vi "GetRangeAndUnits.vi"(0 "Handle":u64, 1 "Controller Channel":i64) -> (7 "FT_Status":u64(ring) items=["FT_OK", "FT_INVALID_HANDLE", "FT_DEVICE_NOT_FOUND", "FT_DEVICE_NOT_OPENED", "FT_IO_ERROR", "FT_INSUFFICIENT_RESOURCES", "FT_INVALID_PARAMETER", "FT_INVALID_BAUD_RATE", "FT_DEVICE_NOT_OPENED_FOR_ERASE", "FT_DEVICE_NOT_OPENED_FOR_WRITE", "FT_FAILED_TO_WRITE_DEVICE", "FT_EEPROM_READ_FAILED", "FT_EEPROM_WRITE_FAILED", "FT_EEPROM_ERASE_FAILED", "FT_EEPROM_NOT_PRESENT", "FT_EEPROM_NOT_PROGRAMMED", "FT_INVALID_ARGS", "FT_NOT_SUPPORTED", "FT_OTHER_ERROR"], 9 "Range":i32, 10 "Range Units":string)   [LabVIEW 2018]
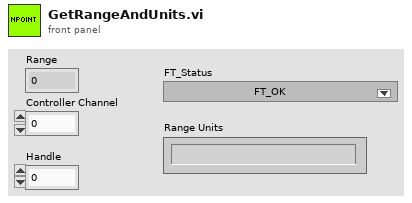
[diagram p1: front panel]
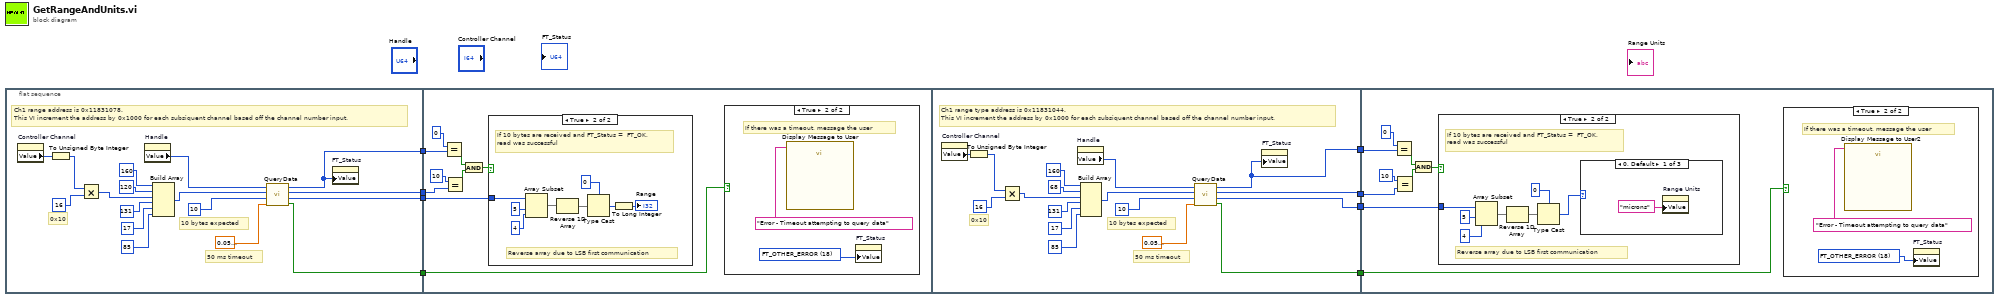
[diagram p0: block diagram]
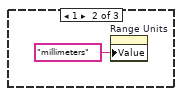
[diagram p6: hidden frame]
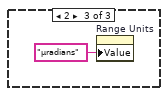
[diagram p7: hidden frame]
diagram:
  n1 = flat-sequence {
    tunnel: [w16] -> w8
    tunnel: [w15] -> w7
    tunnel: [w14] -> w6
    tunnel: [w13] -> w5
    tunnel: w8 -> [w34]
    tunnel: w7 -> [w32]
    tunnel: w6 -> [w31]
    tunnel: w5 -> [w29]
    tunnel: [w48] -> w4
    tunnel: [w52] -> w3
    tunnel: [w51] -> w2
    tunnel: [w50] -> w1
    tunnel: w4 -> [w65]
    tunnel: w3 -> [w62]
    tunnel: w2 -> [w64]
    tunnel: w1 -> [w63]
    frame #0 {
      # "10 bytes expected"
      # "50 ms timeout"
      # "Ch1 range address is 0x11831078.\nThis VI increment the address by 0x1000 for each subsiquent channel based off the channel number input."
      # "0x10"
      n2 = property on="Controller Channel" class="DigNum (strict)"() -> ("Value"=w11:i64)  [unwired: 2 in, 2 out]
      n3 = To Unsigned Byte Integer(number=w11) -> (unsigned 8bit integer=w9:u8)
      n4 = Multiply(x=w9, y=u8 16) -> (x*y=w12:u8)
      n5 = property on="Handle" class="DigNum (strict)"() -> ("Value"=w10:u64)  [unwired: 2 in, 2 out]
      n6 = Build Array(u8 160 ("element"), u8 120 ("element"), w12, u8 131 ("element"), u8 17 ("element"), u8 85 ("element")) -> (w19:u8[])
      n7 = call "QueryData.vi"("TimeoutLengthSeconds"=sgl 0.05, "NumBytesExpected"=u64 10, "Message"=w19, "Handle"=w10) -> ("Timeout"=w14:bool, "Return Array"=w15:u8[], "Bytes Read"=w16:u64, "FT_Status"=w13:u64)  [unwired: 4 in]
      n8 = property on="FT_Status" class="Ring (strict)"("Value"=w13) -> ()  [unwired: 2 in, 2 out]
    }
    frame #1 {
      n9 = Equal?(x=u64 0, y=w29) -> (x = y?=w27:bool)
      n10 = Equal?(x=u64 10, y=w34) -> (x = y?=w28:bool)
      n11 = And(x=w27, y=w28) -> (x .and. y?=w26:bool)
      n12 = case shown="True" w26 {
        tunnel: w32 -> [_ w44]
        frame False {
        }
        frame True {
          # "Reverse array due to LSB first communication"
          # "If 10 bytes are received and FT_Status =  FT_OK,\nread was successful"
          n13 = Array Subset(array=w44, index=5, length=4) -> (w40:u8[])
          n14 = Reverse 1D Array(array=w40) -> (reversed array=w39:u8[])
          n15 = Type Cast(type=0, x=w39) -> (*(type *) &x=w38:i32)
          n16 = To Long Integer(number=w38) -> (32bit integer=→"Range":i32)
        }
      }
      n17 = case shown="True" w31 {
        frame False {
        }
        frame True {
          w35 = u64 18 items=["FT_OK", "FT_INVALID_HANDLE", "FT_DEVICE_NOT_FOUND", "FT_DEVICE_NOT_OPENED", "FT_IO_ERROR", "FT_INSUFFICIENT_RESOURCES", "FT_INVALID_PARAMETER", "FT_INVALID_BAUD_RATE", "FT_DEVICE_NOT_OPENED_FOR_ERASE", "FT_DEVICE_NOT_OPENED_FOR_WRITE", "FT_FAILED_TO_WRITE_DEVICE", "FT_EEPROM_READ_FAILED", "FT_EEPROM_WRITE_FAILED", "FT_EEPROM_ERASE_FAILED", "FT_EEPROM_NOT_PRESENT", "FT_EEPROM_NOT_PROGRAMMED", "FT_INVALID_ARGS", "FT_NOT_SUPPORTED", "FT_OTHER_ERROR"] ("FT_Status")
          # "If there was a timeout, message the user"
          n18 = call "Display Message to User"("Message"="Error - Timeout attempting to query data") -> ()  [unwired: 9 in, 2 out]
          n19 = property on="FT_Status" class="Ring (strict)"("Value"=w35) -> ()  [unwired: 2 in, 2 out]
        }
      }
    }
    frame #2 {
      # "10 bytes expected"
      # "50 ms timeout"
      # "Ch1 range type address is 0x11831044.\nThis VI increment the address by 0x1000 for each subsiquent channel based off the channel number input."
      # "0x10"
      n20 = property on="Controller Channel" class="DigNum (strict)"() -> ("Value"=w47:i64)  [unwired: 2 in, 2 out]
      n21 = To Unsigned Byte Integer(number=w47) -> (unsigned 8bit integer=w45:u8)
      n22 = Multiply(x=w45, y=u8 16) -> (x*y=w49:u8)
      n23 = property on="Handle" class="DigNum (strict)"() -> ("Value"=w46:u64)  [unwired: 2 in, 2 out]
      n24 = Build Array(u8 160 ("element"), u8 68 ("element"), w49, u8 131 ("element"), u8 17 ("element"), u8 85 ("element")) -> (w55:u8[])
      n25 = call "QueryData.vi"("TimeoutLengthSeconds"=sgl 0.05, "NumBytesExpected"=u64 10, "Message"=w55, "Handle"=w46) -> ("Timeout"=w50:bool, "Return Array"=w51:u8[], "Bytes Read"=w52:u64, "FT_Status"=w48:u64)  [unwired: 4 in]
      n26 = property on="FT_Status" class="Ring (strict)"("Value"=w48) -> ()  [unwired: 2 in, 2 out]
    }
    frame #3 {
      n27 = Equal?(x=u64 0, y=w65) -> (x = y?=w67:bool)
      n28 = Equal?(x=u64 10, y=w62) -> (x = y?=w68:bool)
      n29 = And(x=w67, y=w68) -> (x .and. y?=w66:bool)
      n30 = case shown="True" w66 {
        tunnel: w64 -> [_ w79]
        frame False {
        }
        frame True {
          # "Reverse array due to LSB first communication"
          # "If 10 bytes are received and FT_Status =  FT_OK,\nread was successful"
          n31 = Array Subset(array=w79, index=5, length=4) -> (w75:u8[])
          n32 = Reverse 1D Array(array=w75) -> (reversed array=w74:u8[])
          n33 = Type Cast(type=0, x=w74) -> (*(type *) &x=w73:i32)
          n34 = case shown="0, Default" w73 {
            frame 0, Default {
              n35 = property on="Range Units" class="Str"("Value"="microns" ("Range Units")) -> ()  [unwired: 2 in, 2 out]
            }
            frame 1 {
              n36 = property on="Range Units" class="Str"("Value"="millimeters" ("Range Units")) -> ()  [unwired: 2 in, 2 out]
            }
            frame 2 {
              n37 = property on="Range Units" class="Str"("Value"="µradians" ("Range Units")) -> ()  [unwired: 2 in, 2 out]
            }
          }
        }
      }
      n38 = case shown="True" w63 {
        frame False {
        }
        frame True {
          w71 = u64 18 items=["FT_OK", "FT_INVALID_HANDLE", "FT_DEVICE_NOT_FOUND", "FT_DEVICE_NOT_OPENED", "FT_IO_ERROR", "FT_INSUFFICIENT_RESOURCES", "FT_INVALID_PARAMETER", "FT_INVALID_BAUD_RATE", "FT_DEVICE_NOT_OPENED_FOR_ERASE", "FT_DEVICE_NOT_OPENED_FOR_WRITE", "FT_FAILED_TO_WRITE_DEVICE", "FT_EEPROM_READ_FAILED", "FT_EEPROM_WRITE_FAILED", "FT_EEPROM_ERASE_FAILED", "FT_EEPROM_NOT_PRESENT", "FT_EEPROM_NOT_PROGRAMMED", "FT_INVALID_ARGS", "FT_NOT_SUPPORTED", "FT_OTHER_ERROR"] ("FT_Status")
          # "If there was a timeout, message the user"
          n39 = call "Display Message to User2"("Message"="Error - Timeout attempting to query data") -> ()  [unwired: 9 in, 2 out]
          n40 = property on="FT_Status" class="Ring (strict)"("Value"=w71) -> ()  [unwired: 2 in, 2 out]
        }
      }
    }
  }
